vi "mouse_position.vi"(1 "Object":refnum<vi>, 2 "Pane":refnum<vi>, 3 "VI":refnum<vi>) -> (0 "Mouse position relative to object":cluster{"X":i32, "Y":i32})   [LabVIEW 2017]
uses:
  <vilib>/Utility/inputDevices.llb/mouseAcquire.vi
panel:
  # "This VI takes a parent VI, a pane from that VI, and an object from that pane, and tells the position of the mouse on that object."
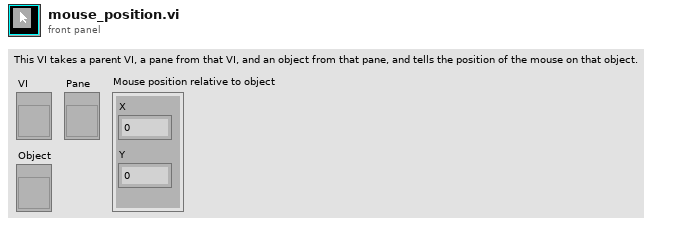
[diagram p1: front panel]
types:
  T1 = typedef "LVRectTypeDef.ctl" = cluster{"Left":i16, "Top":i16, "Right":i16, "Bottom":i16}
  T2 = typedef "LVPointTypeDef.ctl" = cluster{"Horizontal":i16, "Vertical":i16}
  T3 = typedef "LVPositionTypeDef.ctl" = cluster{"Left":i32, "Top":i32}
  T4 = cluster{"Horizontal":i32, "Vertical":i32, "Scrolling":i32}
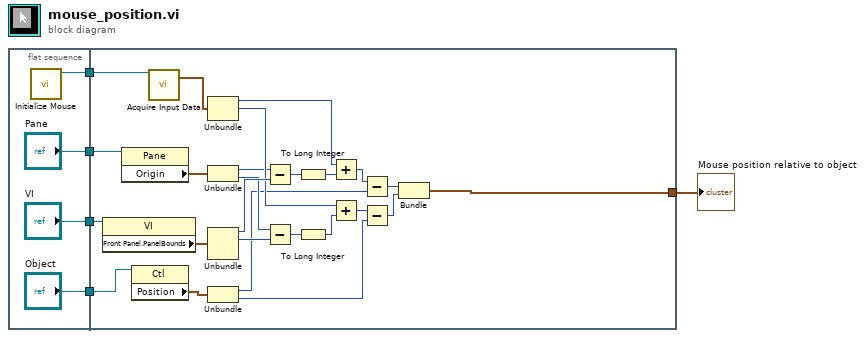
[diagram p0: block diagram]
diagram:
  n1 = flat-sequence {
    tunnel: [w9] -> w5
    tunnel: ["Pane"] -> w4
    tunnel: ["VI"] -> w3
    tunnel: ["Object"] -> w2
    tunnel: w5 -> [w17]
    tunnel: w4 -> [w16]
    tunnel: w3 -> [w15]
    tunnel: w2 -> [w11]
    tunnel: [w10] -> w1
    frame #0 {
      n2 = call <vilib>:"Initialize Mouse.vi"() -> ("device ID"=w9:refnum<k1>)  [unwired: 10 in, 1 out]
    }
    frame #1 {
      n3 = property class="VI"(reference=w15) -> ("Front Panel.PanelBounds"=w33:T1)  [unwired: 1 in, 2 out]
      n4 = property class="Pane"(reference=w16) -> ("Origin"=w32:T2)  [unwired: 1 in, 2 out]
      n5 = property class="Ctl"(reference=w11) -> ("Position"=w12:T3)  [unwired: 1 in, 2 out]
      n6 = call-poly <vilib>:"Acquire Input Data.vi"("device ID"=w17) -> ("axis info"=w34:T4)  [unwired: 15 in, 3 out]
      n7 = Unbundle(w34) -> ("Horizontal"=w29:i32, "Vertical"=w28:i32)  [unwired: 1 out]
      n8 = Unbundle(w32) -> ("Horizontal"=w18:i16, "Vertical"=w19:i16)
      n9 = Unbundle(w33) -> ("Left"=w31:i16, "Top"=w30:i16)  [unwired: 2 out]
      n10 = Unbundle(w12) -> ("Left"=w14:i32, "Top"=w13:i32)
      n11 = Subtract(x=w18, y=w31) -> (x-y=w26:i16)
      n12 = Subtract(x=w19, y=w30) -> (x-y=w25:i16)
      n13 = To Long Integer(number=w26) -> (32bit integer=w27:i32)
      n14 = To Long Integer(number=w25) -> (32bit integer=w24:i32)
      n15 = Add(x=w29, y=w27) -> (x+y=w23:i32)
      n16 = Add(x=w28, y=w24) -> (x+y=w22:i32)
      n17 = Subtract(x=w23, y=w14) -> (x-y=w21:i32)
      n18 = Subtract(x=w22, y=w13) -> (x-y=w20:i32)
      n19 = Bundle(w21, w20) -> (w10:cluster{i32, i32})  [unwired: 1 in]
    }
  }
  "Mouse position relative to object" <- w1
